vi "Conv_AngleRadians_Heading.vi"(10 "Radians":dbl) -> (2 "Heading":dbl)   [LabVIEW 2019, in "Trajectory_Library.lvlib"]
doc: "Convert angle (radians) to heading (+/- PI ) (radians)\nNOTE: increases counter clockwise"
uses:
  Trajectory_Library.lvlib
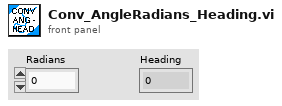
[diagram p1: front panel]
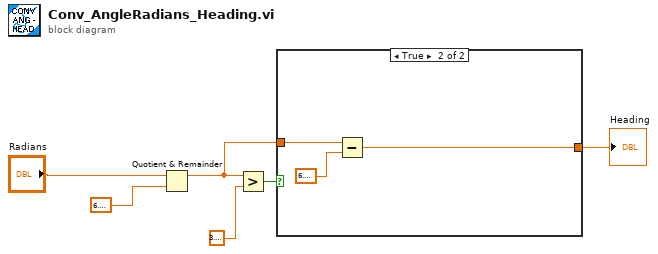
[diagram p0: block diagram]
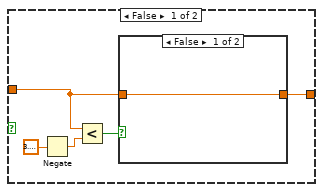
[diagram p2: hidden frame]
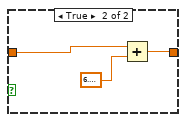
[diagram p3: hidden frame]
diagram:
  n1 = Quotient & Remainder(x="Radians", y=6.283185307179586) -> (x-y*floor(x/y)=w2:dbl)  [unwired: 1 out]
  n2 = Greater?(x=w2, y=3.141592653589793) -> (0:w3:bool)
  n3 = case shown="True" w3 {
    tunnel: w2 -> [w8 w17]
    tunnel: [w7 w16] -> w1
    frame False {
      n4 = Negate(x=3.141592653589793) -> (-x=w10:dbl)
      n5 = Less?(x=w8, y=w10) -> (x < y?=w9:bool)
      n6 = case shown="False" w9 {
        tunnel: w8 -> [w12 w13]
        tunnel: [w12 w14] -> w7
        frame False {
        }
        frame True {
          n7 = Add(x=w13, y=6.283185307179586) -> (x+y=w14:dbl)
        }
      }
    }
    frame True {
      n8 = Subtract(x=w17, y=6.283185307179586) -> (x-y=w16:dbl)
    }
  }
  "Heading" <- w1
